vi "encoder_debug_v2.vi"() -> ()   [LabVIEW 2014]
uses:
  <vilib>/rvi/Emulation/niFpgaGetClockAttributes.vi
  <vilib>/rvi/Emulation/niFpgaSctlEmulationGetInTimedLoop.vi
  <vilib>/rvi/Emulation/niFpgaEmulationReportErrorSimple.vi
  <vilib>/rvi/Emulation/niFpgaProcessEmulError.vi
  <vilib>/rvi/interface/RandomDataEmulation/nirviRandomDataMultiElementFPGAFIFO.vi
  <instcachedir>/0/nirviRandomDataMultiElementFPGAFIFO_AD0CFC12EF974623A9C2E4184BC062B2.lvgen/nirviRandomDataMultiElementFPGAFIFO_AD0CFC12EF974623A9C2E4184BC062B2_010.vi
  <vilib>/rvi/interface/RandomDataEmulation/niFpgaRandomDataHandleErrors.vi
  <vilib>/rvi/Emulation/niFpgaCriticalErrorInLSC.vi
  <vilib>/rvi/eio/common/nirviEmuTemplateMethod_errors.vi
  <vilib>/rvi/DataTransferAndStorage/Container/XNode/niFpgaContainer.xnode
  <vilib>/rvi/interface/RandomDataEmulation/nirviRandomDataFpgaMultiElementTemplate.vi
  <vilib>/eio/EIONode/EIONode.xnode
  <vilib>/rvi/Analysis/measure/butterworth/XNode/niFpgaButterworthFilter.xnode
panel:
  in  "Stop motor":bool
  out "omega_p2 (rad/s)":fxp<+/-,36,13>
  out "Dp2_d (mm/s)":fxp<+/-,36,13>
  out "omega_p2 (Mavg)":fxp<+/-,36,14>
  out "Dp2_d (Mavg)":fxp<+/-,36,14>
  in  "mt0_p2":u32
  out "Dp2_d (Mavg w. f.)":fxp<+/-,36,14>
  out "Dp1_d (Mavg w. f.)":fxp<+/-,36,14>
  in  "Dp_d (Mavg) coeff.":i32[](array[numeric])=[946630756, 63555534]
  in  "Dy_d (Mavg) coeff.":i32[](array[numeric])=[946630756, 63555534]
  out "omega_p2 (Mavg w. f.)":fxp<+/-,36,14>
  in  "omega_y(Mavg) coeff.":i32[](array[numeric])=[946630756, 63555534]
  out "omega_p1 (Mavg w. f)":fxp<+/-,36,14>
  in  "omega_P(Mavg) coeff.":i32[](array[numeric])=[946630756, 63555534]
  out "Dp1_d (T)":fxp<+/-,36,13>
  out "omega_p1 (T)":fxp<+/-,36,13>
  out "Dp2_d (T)":fxp<+/-,36,13>
  out "omega_p2 (T)":fxp<+/-,36,13>
  out "mt_omega_p2":u32
  out "Encoder Position_p2":i32
  out "D_p2":fxp<+/-,32,7>
  out "rad_p2":fxp<+/-,36,15>
  out "D_p1":fxp<+/-,32,7>
  out "rad_p1":fxp<+/-,36,15>
  out "Encoder Position_p1":i32
  out "Dp1_d (Mavg)":fxp<+/-,36,14>
  out "omega_p1 (Mavg)":fxp<+/-,36,14>
  in  "Dp_d_M_avg_Tc (uSec)":i32
  in  "Vp. Est.":i16(ring) items=["T", "Mavg", "Mavg w. f."]
  in  "Mag. factor_p":fxp<+/-,20,3>
  in  "Belt_out_p":fxp<+/-,7,7>
  in  "Belt_in_p":fxp<+/-,6,6>
  in  "mt0_p1":u32
  out "Dp1_d (mm/s)":fxp<+/-,36,13>
  out "omega_p1 (rad/s)":fxp<+/-,36,13>
  out "mt_omega_p1":u32
  in  "Encoder reset_p":bool
  out "Time now(s)":fxp<+,52,14>
  in  "Ini coe.":bool
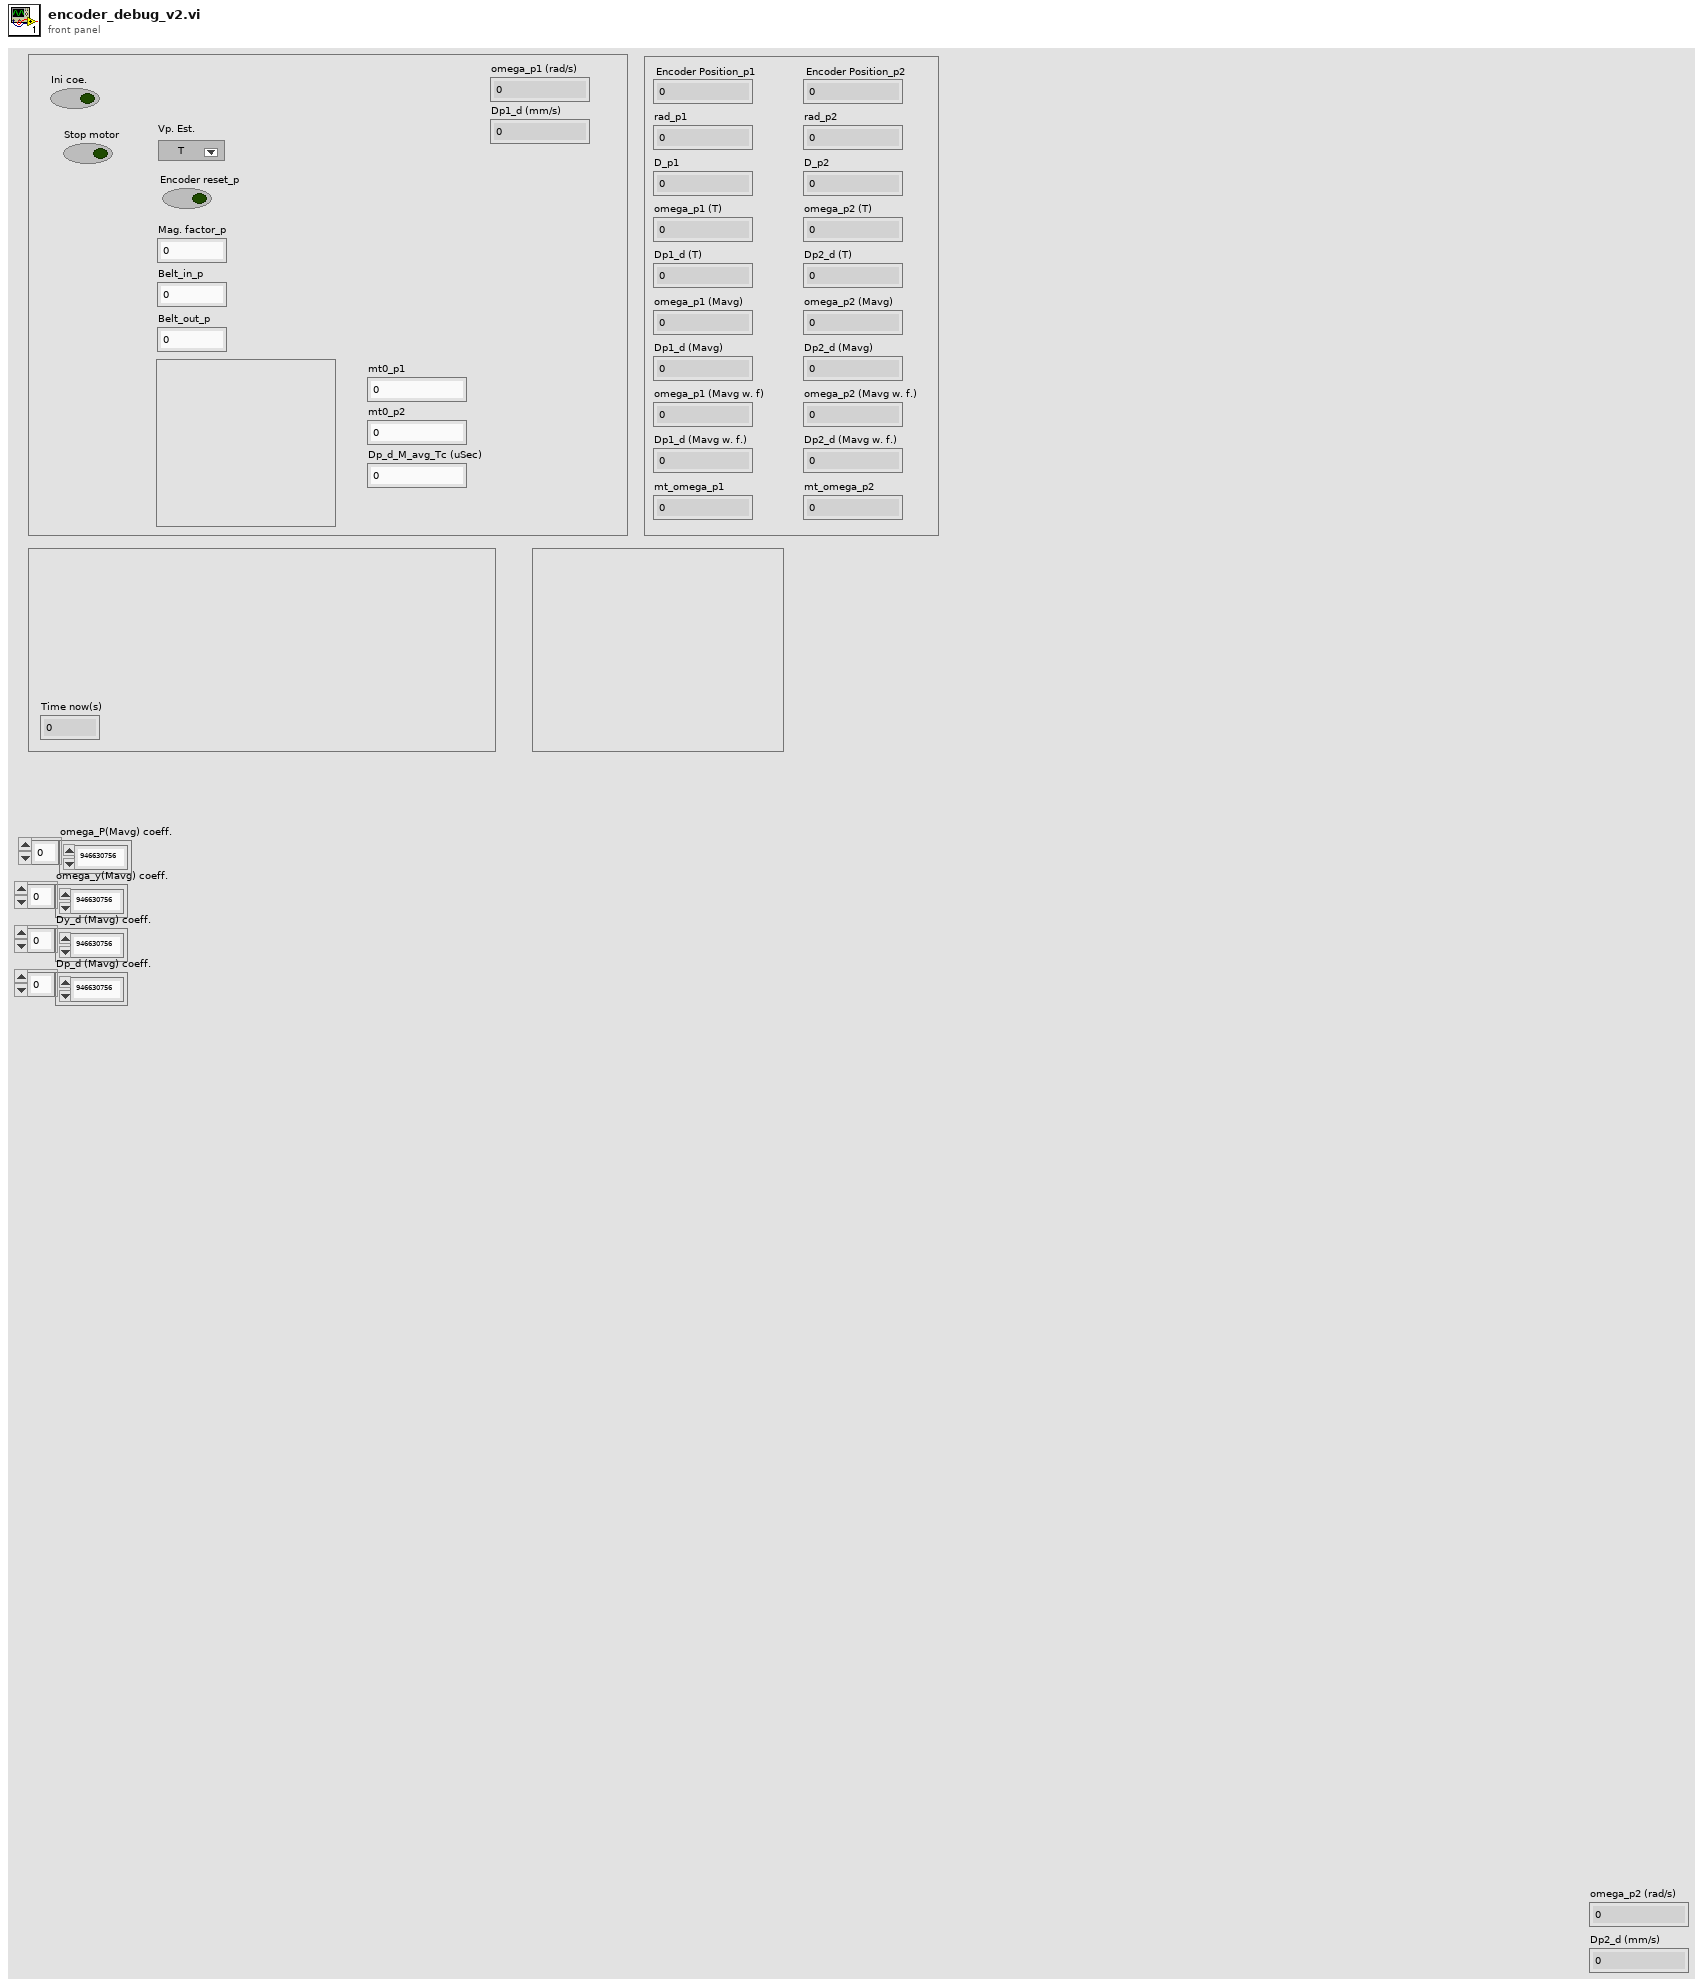
[diagram p1: front panel]
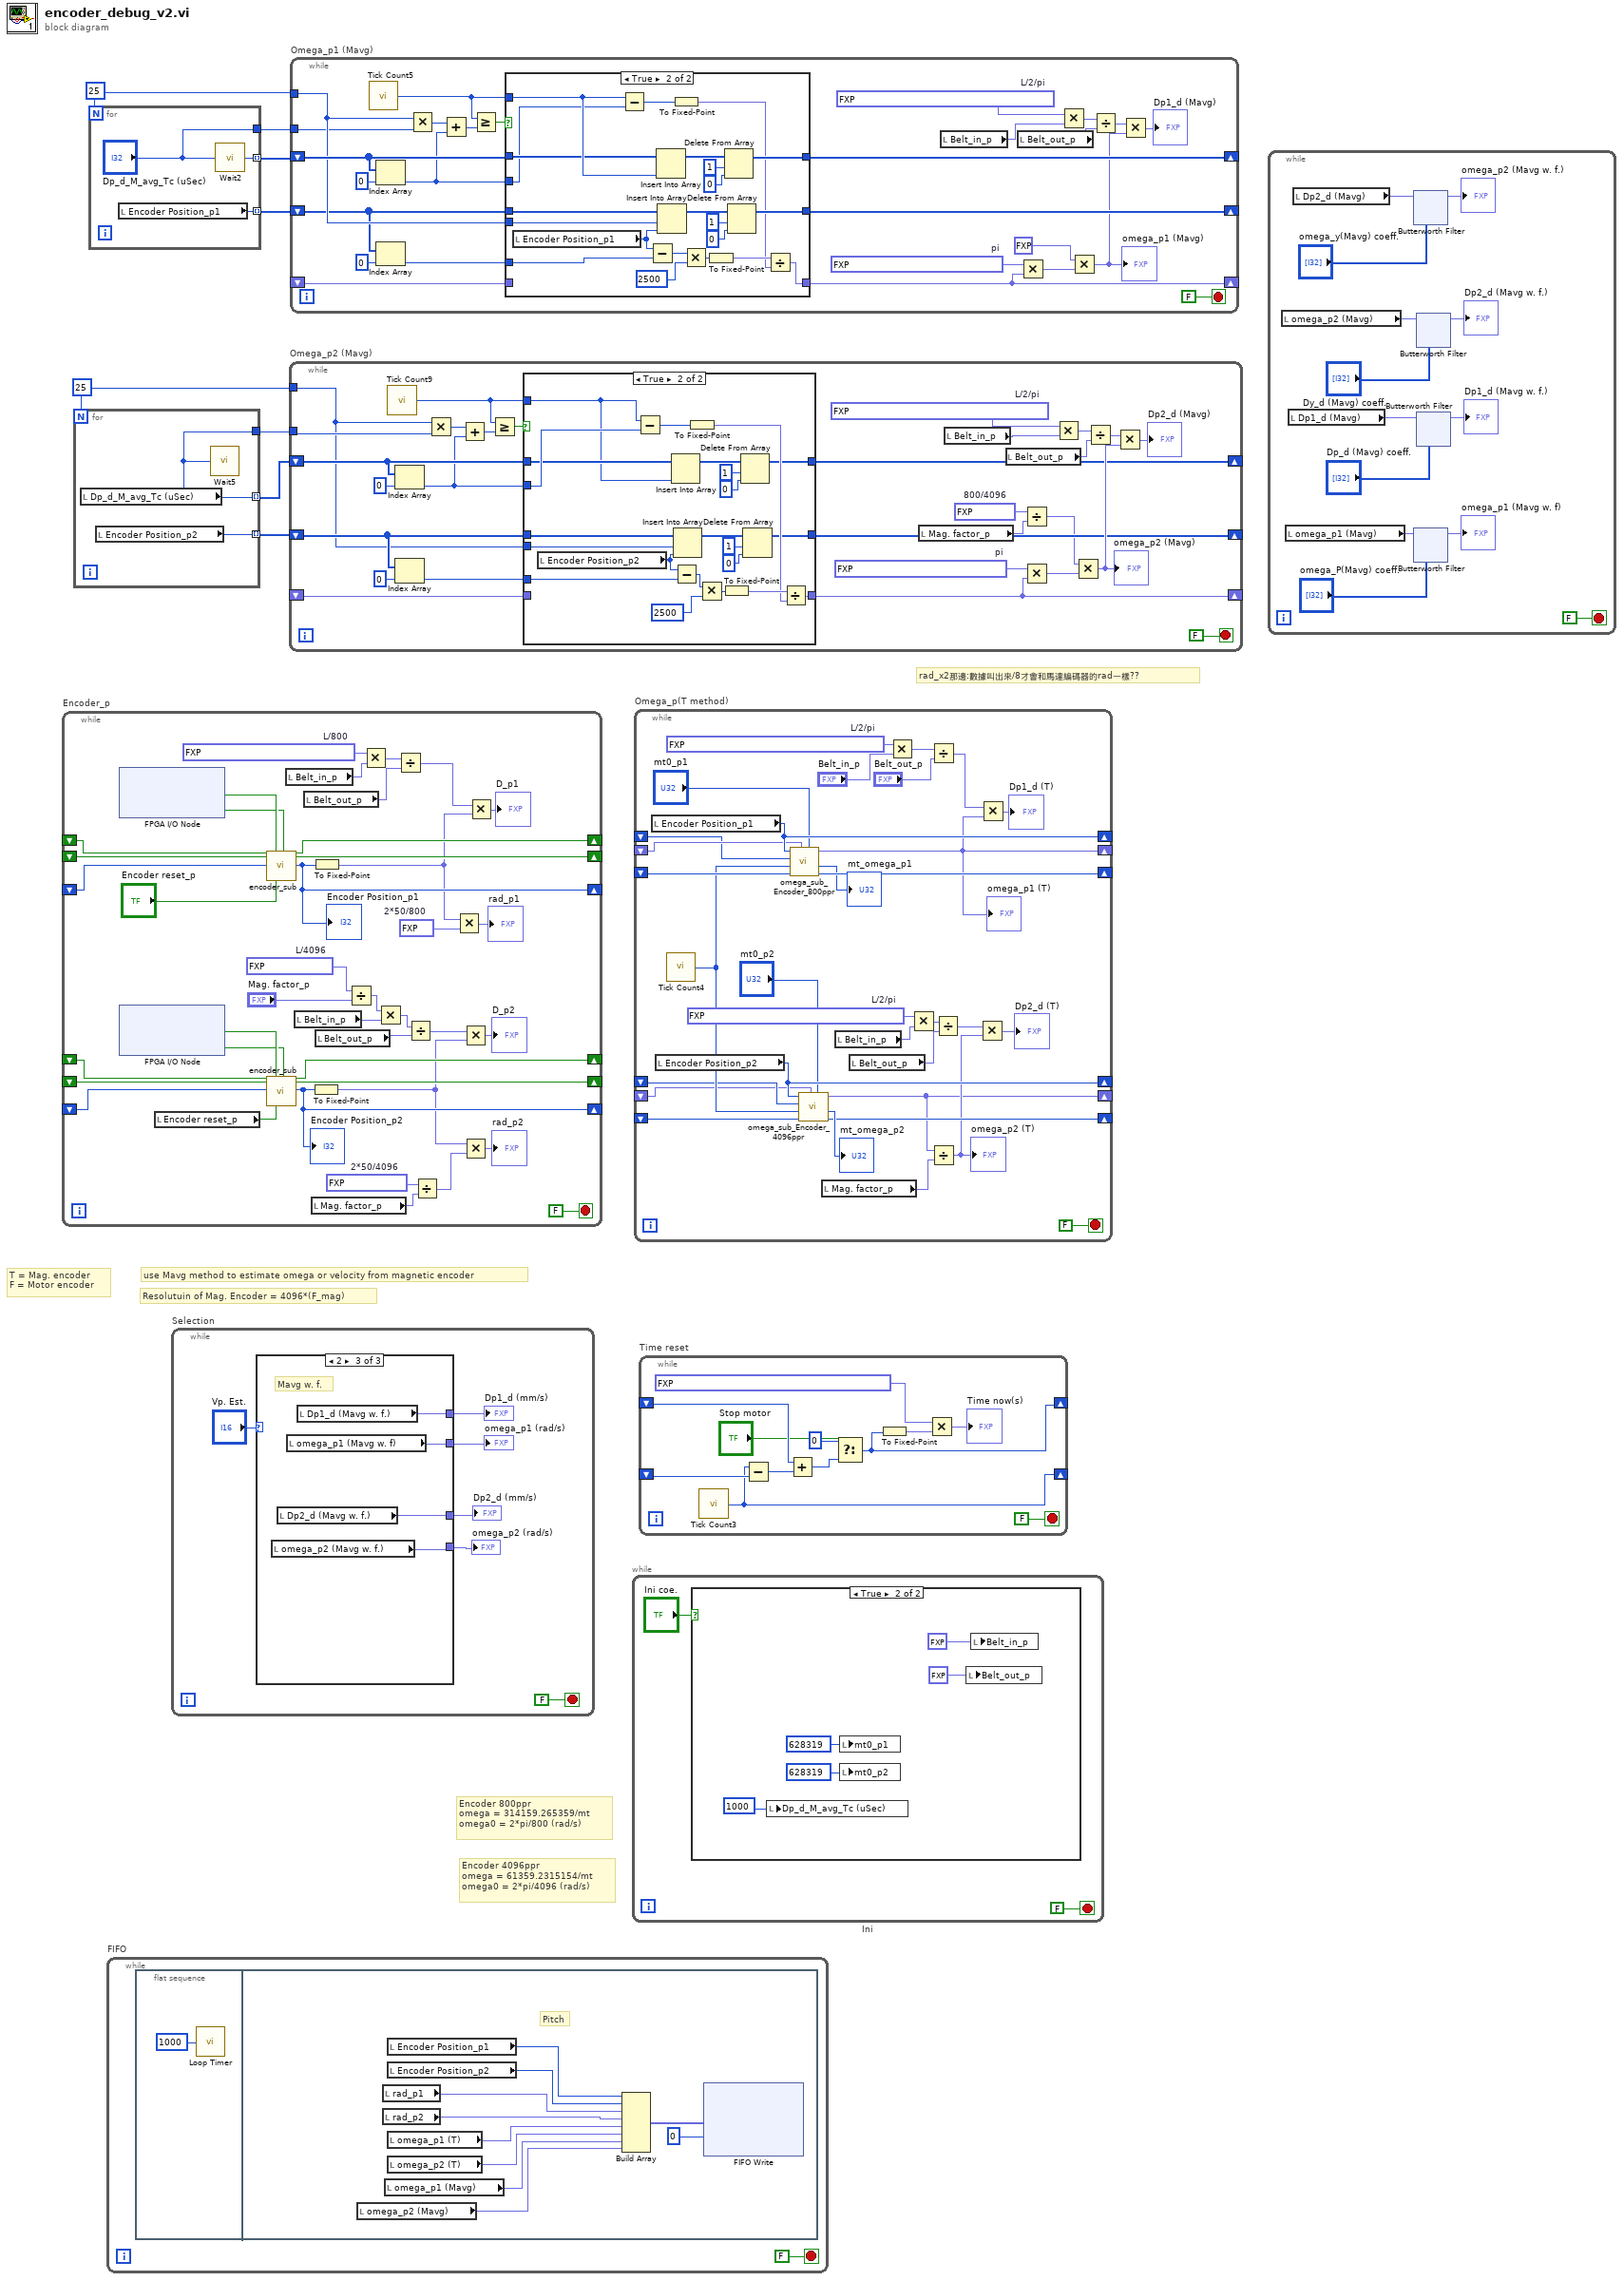
[diagram p0: block diagram]
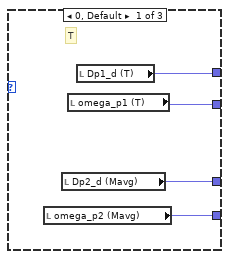
[diagram p4: hidden frame]
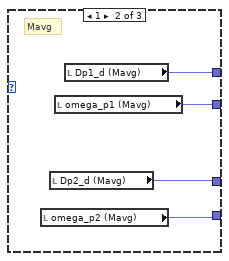
[diagram p5: hidden frame]
diagram:
  w2 = 25
  w8 = 25
  # "T = Mag. encoder\nF = Motor encoder"
  # "rad_x2那邊:數據叫出來/8才會和馬達編碼器的rad一樣??"
  # "Encoder 4096ppr\nomega = 61359.2315154/mt\nomega0 = 2*pi/4096 (rad/s)"
  # "Encoder 800ppr\nomega = 314159.265359/mt\nomega0 = 2*pi/800 (rad/s)"
  # "Resolutuin of Mag. Encoder = 4096*(F_mag)"
  # "use Mavg method to estimate omega or velocity from magnetic encoder"
  n1 = while "Encoder_p" {
    shift-right: [w46] -> _
    shift-left: _ -> [w45]
    shift-right: [w47] -> _
    shift-left: _ -> [w44]
    shift-right: [w41] -> _
    shift-left: _ -> [w43]
    shift-right: [w32] -> _
    shift-left: _ -> [w31]
    shift-right: [w33] -> _
    shift-left: _ -> [w34]
    shift-right: [w28] -> _
    shift-left: _ -> [w29]
    stop <- FALSE stop-if-true
    w24 = fxp<+/-,20,-5> 0.00048828125  # L/4096
    w22 = fxp<+/-,16,1> 0.0244140625  # 2*50/4096
    w40 = fxp<+/-,20,-5> 0.002499997615814209  # L/800
    w14 = fxp<+/-,16,1> 0.125  # 2*50/800
    n2 = xnode "FPGA I/O Node"() -> ("Mod7/DIO0"=w49:bool, "Mod7/DIO1"=w48:bool)  [unwired: 2 in, 2 out]
    n3 = xnode "FPGA I/O Node"() -> ("Mod7/DIO4"=w36:bool, "Mod7/DIO5"=w35:bool)  [unwired: 2 in, 2 out]
    n4 = local read "Encoder reset_p"() -> (w30:bool)
    n5 = call "encoder_sub.vi"("A_pre"=w45, "B_pre"=w44, "Encoder Position_pre"=w43, "A input"=w49, "Encoder Position Reset"="Encoder reset_p", "B input"=w48) -> ("A"=w46:bool, "B"=w47:bool, "Encoder Position (Counts)"=w41:i32)  [unwired: 19 in]
    "Encoder Position_p1" <- w41
    n6 = call "encoder_sub.vi"("A_pre"=w31, "B_pre"=w34, "Encoder Position_pre"=w29, "A input"=w36, "Encoder Position Reset"=w30, "B input"=w35) -> ("A"=w32:bool, "B"=w33:bool, "Encoder Position (Counts)"=w28:i32)  [unwired: 19 in]
    "Encoder Position_p2" <- w28
    n7 = local read "Belt_in_p"() -> (w39:fxp<+/-,6,6>)
    n8 = local read "Belt_in_p"() -> (w25:fxp<+/-,6,6>)
    n9 = local read "Belt_out_p"() -> (w37:fxp<+/-,7,7>)
    n10 = local read "Mag. factor_p"() -> (w21:fxp<+/-,20,3>)
    n11 = To Fixed-Point(number=w28) -> (fixed-point=w10:fxp<+/-,32,32>)  [unwired: 1 in]
    n12 = To Fixed-Point(number=w41) -> (fixed-point=w15:fxp<+/-,32,32>)  [unwired: 1 in]
    n13 = local read "Belt_out_p"() -> (w27:fxp<+/-,7,7>)
    n14 = Divide(x=w24, y="Mag. factor_p") -> (x/y=w23:fxp<+/-,41,13>)
    n15 = Multiply(x=w40, y=w39) -> (x*y=w38:fxp<+/-,26,1>)
    n16 = Multiply(x=w23, y=w25) -> (x*y=w26:fxp<+/-,46,18>)
    n17 = Divide(x=w38, y=w37) -> (x/y=w17:fxp<+/-,33,1>)
    n18 = Divide(x=w26, y=w27) -> (x/y=w12:fxp<+/-,53,18>)
    n19 = Divide(x=w22, y=w21) -> (x/y=w9:fxp<+/-,37,19>)
    n20 = Multiply(x=w15, y=w14) -> (x*y=→"rad_p1":fxp<+/-,48,33>)
    n21 = Multiply(x=w12, y=w10) -> (x*y=→"D_p2":fxp<+/-,64,49>)
    n22 = Multiply(x=w10, y=w9) -> (x*y=→"rad_p2":fxp<+/-,64,50>)
    n23 = Multiply(x=w17, y=w15) -> (x*y=→"D_p1":fxp<+/-,64,32>)
  }
  n24 = for {
    N: w2 -> [_]
    tunnel: [w51] -> w4 mode=indexing
    tunnel: [w50] -> w3 mode=indexing
    tunnel: [w50] -> w1
    n25 = local read "Dp_d_M_avg_Tc (uSec)"() -> (w50:i32)
    n26 = local read "Encoder Position_p2"() -> (w51:i32)
    n27 = call "Wait5"("Count(uSec)"=w50) -> ()  [unwired: 1 out]
  }
  n28 = for {
    N: w8 -> [_]
    tunnel: ["Dp_d_M_avg_Tc (uSec)"] -> w5
    tunnel: [w53] -> w7 mode=indexing
    tunnel: [w52] -> w6 mode=indexing
    n29 = local read "Encoder Position_p1"() -> (w52:i32)
    n30 = call "Wait2"("Count(uSec)"="Dp_d_M_avg_Tc (uSec)") -> ("Tick Count(uSec)"=w53:u32)
  }
  n31 = while "FIFO" {
    stop <- FALSE stop-if-true
    n32 = flat-sequence {
      frame #0 {
        n33 = call "Loop Timer"("Count(uSec)"=u32 1000) -> ()  [unwired: 1 out]
      }
      frame #1 {
        # "Pitch"
        n34 = local read "omega_p2 (Mavg)"() -> (w57:fxp<+/-,36,14>)
        n35 = local read "rad_p1"() -> (w64:fxp<+/-,36,15>)
        n36 = local read "rad_p2"() -> (w63:fxp<+/-,36,15>)
        n37 = local read "omega_p1 (Mavg)"() -> (w61:fxp<+/-,36,14>)
        n38 = local read "Encoder Position_p1"() -> (w66:i32)
        n39 = local read "Encoder Position_p2"() -> (w65:i32)
        n40 = local read "omega_p1 (T)"() -> (w59:fxp<+/-,36,13>)
        n41 = local read "omega_p2 (T)"() -> (w60:fxp<+/-,36,13>)
        n42 = Build Array(w66, w65, w64, w63, w59, w60, w61, w57) -> (w58:fxp<+/-,55,32>[])
        n43 = xnode ("FIFO Write")("Element"=w58, "Timeout"=0) -> ()  [unwired: 1 in, 2 out]
      }
    }
  }
  n44 = while "Selection" {
    stop <- FALSE stop-if-true
    n45 = case shown="2" "Vp. Est." {
      tunnel: [w76 w79 w84] -> w71
      tunnel: [w75 w80 w83] -> w72
      tunnel: [w74 w77 w81] -> w69
      tunnel: [w73 w78 w82] -> w68
      frame 0, Default {
        # "T"
        n46 = local read "omega_p2 (Mavg)"() -> (w74:fxp<+/-,36,14>)
        n47 = local read "Dp2_d (Mavg)"() -> (w73:fxp<+/-,36,14>)
        n48 = local read "omega_p1 (T)"() -> (w76:fxp<+/-,36,13>)
        n49 = local read "Dp1_d (T)"() -> (w75:fxp<+/-,36,13>)
      }
      frame 1 {
        # "Mavg"
        n50 = local read "omega_p2 (Mavg)"() -> (w77:fxp<+/-,36,14>)
        n51 = local read "Dp2_d (Mavg)"() -> (w78:fxp<+/-,36,14>)
        n52 = local read "omega_p1 (Mavg)"() -> (w79:fxp<+/-,36,14>)
        n53 = local read "Dp1_d (Mavg)"() -> (w80:fxp<+/-,36,14>)
      }
      frame 2 {
        # "Mavg w. f."
        n54 = local read "omega_p2 (Mavg w. f.)"() -> (w81:fxp<+/-,36,14>)
        n55 = local read "Dp2_d (Mavg w. f.)"() -> (w82:fxp<+/-,36,14>)
        n56 = local read "omega_p1 (Mavg w. f)"() -> (w84:fxp<+/-,36,14>)
        n57 = local read "Dp1_d (Mavg w. f.)"() -> (w83:fxp<+/-,36,14>)
      }
    }
    "Dp1_d (mm/s)" <- w72
    "omega_p1 (rad/s)" <- w71
    "Dp2_d (mm/s)" <- w68
    "omega_p2 (rad/s)" <- w69
  }
  n58 = while "Omega_p2 (Mavg)" {
    shift-right: [w86] -> _
    shift-left: w4 -> [w107]
    shift-right: [w87] -> _
    shift-left: w3 -> [w105]
    shift-right: [w91] -> _
    shift-left: _ -> [w89]
    tunnel: w2 -> [w103]
    tunnel: w1 -> [w108]
    stop <- FALSE stop-if-true
    w92 = fxp<+/-,27,3> 3.1415926814079285  # pi
    w95 = fxp<+,32,0> 0.1953125  # 800/4096
    w100 = fxp<+/-,32,0> 0.3183098859153688  # L/2/pi
    n59 = call "Tick Count9"() -> ("Tick Count(uSec)"=w102:u32)
    n60 = Index Array(array=w105, index=0) -> (element=w104:i32)
    n61 = Index Array(array=w107, index=0) -> (element=w106:i32)
    n62 = Multiply(x=w103, y=w108) -> (x*y=w111:i32)
    n63 = Add(x=w111, y=w104) -> (x+y=w110:i32)
    n64 = Greater Or Equal?(x=w102, y=w110) -> (x >= y?=w109:bool)
    n65 = case shown="True" w109 {
      tunnel: w107 -> [w115 w130]
      tunnel: w106 -> [_ w122]
      tunnel: w105 -> [w116 w131]
      tunnel: w104 -> [_ w132]
      tunnel: w103 -> [_ w129]
      tunnel: w102 -> [_ w117]
      tunnel: [w115 w120] -> w86
      tunnel: [w116 w119] -> w87
      tunnel: [w114 w118] -> w91
      tunnel: w89 -> [w114 _]
      frame False {
      }
      frame True {
        n66 = local read "Encoder Position_p2"() -> (w121:i32)
        n67 = Subtract(x=w117, y=w132) -> (x-y=w133:u32)
        n68 = Insert Into Array(array=w131, new element=w117) -> (w135:i32[])  [unwired: 1 in]
        n69 = Subtract(x=w121, y=w122) -> (x-y=w126:i32)
        n70 = Insert Into Array(array=w130, index=w129, new element=w121) -> (w136:i32[])
        n71 = To Fixed-Point(number=w133) -> (fixed-point=w123:fxp<+,32,32>)  [unwired: 1 in]
        n72 = Multiply(x=w126, y=2500) -> (x*y=w127:i32)
        n73 = To Fixed-Point(number=w127) -> (fixed-point=w128:fxp<+/-,32,32>)  [unwired: 1 in]
        n74 = Delete From Array(array=w135, length=1, index=0) -> (array with subset deleted=w119:i32[])  [unwired: 1 out]
        n75 = Delete From Array(array=w136, length=1, index=0) -> (array with subset deleted=w120:i32[])  [unwired: 1 out]
        n76 = Divide(x=w128, y=w123) -> (x/y=w118:fxp<+/-,64,32>)
      }
    }
    n77 = local read "Mag. factor_p"() -> (w94:fxp<+/-,20,3>)
    n78 = local read "Belt_in_p"() -> (w97:fxp<+/-,6,6>)
    n79 = local read "Belt_out_p"() -> (w96:fxp<+/-,7,7>)
    n80 = Divide(x=w95, y=w94) -> (x/y=w85:fxp<+/-,32,1>)
    n81 = Multiply(x=w92, y=w91) -> (x*y=w93:fxp<+/-,64,35>)
    n82 = Multiply(x=w100, y=w97) -> (x*y=w101:fxp<+/-,38,6>)
    n83 = Multiply(x=w85, y=w93) -> (x*y=w88:fxp<+/-,64,36>)
    "omega_p2 (Mavg)" <- w88
    n84 = Divide(x=w101, y=w96) -> (x/y=w99:fxp<+/-,45,6>)
    n85 = Multiply(x=w99, y=w88) -> (x*y=→"Dp2_d (Mavg)":fxp<+/-,64,41>)
  }
  n86 = while "Omega_p1 (Mavg)" {
    tunnel: w8 -> [w157]
    shift-right: [w155] -> _
    shift-left: w7 -> [w160]
    shift-right: [w154] -> _
    shift-left: w6 -> [w156]
    shift-right: [w153] -> _
    shift-left: _ -> [w152]
    tunnel: w5 -> [w150]
    stop <- FALSE stop-if-true
    w144 = fxp<+/-,27,3> 3.1415926814079285  # pi
    w143 = fxp<+/-,32,0> 0.3183098859153688  # L/2/pi
    n87 = call "Tick Count5"() -> ("Tick Count(uSec)"=w161:u32)
    n88 = Index Array(array=w160, index=0) -> (element=w159:u32)
    n89 = Index Array(array=w156, index=0) -> (element=w158:i32)
    n90 = Multiply(x=w157, y=w150) -> (x*y=w163:i32)
    n91 = Add(x=w163, y=w159) -> (x+y=w162:u32)
    n92 = Greater Or Equal?(x=w161, y=w162) -> (x >= y?=w151:bool)
    n93 = case shown="True" w151 {
      tunnel: w161 -> [_ w184]
      tunnel: w157 -> [_ w181]
      tunnel: w160 -> [w168 w183]
      tunnel: w159 -> [_ w182]
      tunnel: w158 -> [_ w178]
      tunnel: w156 -> [w167 w180]
      tunnel: [w166 w176] -> w153
      tunnel: [w168 w175] -> w155
      tunnel: [w167 w174] -> w154
      tunnel: w152 -> [w166 _]
      frame False {
      }
      frame True {
        n94 = local read "Encoder Position_p1"() -> (w177:i32)
        n95 = Subtract(x=w184, y=w182) -> (x-y=w185:u32)
        n96 = Subtract(x=w177, y=w178) -> (x-y=w170:i32)
        n97 = Insert Into Array(array=w183, new element=w184) -> (w187:u32[])  [unwired: 1 in]
        n98 = Insert Into Array(array=w180, index=w181, new element=w177) -> (w188:i32[])
        n99 = To Fixed-Point(number=w185) -> (fixed-point=w172:fxp<+,32,32>)  [unwired: 1 in]
        n100 = Multiply(x=w170, y=2500) -> (x*y=w171:i32)
        n101 = To Fixed-Point(number=w171) -> (fixed-point=w179:fxp<+/-,32,32>)  [unwired: 1 in]
        n102 = Delete From Array(array=w187, length=1, index=0) -> (array with subset deleted=w175:u32[])  [unwired: 1 out]
        n103 = Delete From Array(array=w188, length=1, index=0) -> (array with subset deleted=w174:i32[])  [unwired: 1 out]
        n104 = Divide(x=w179, y=w172) -> (x/y=w176:fxp<+/-,64,32>)
      }
    }
    n105 = local read "Belt_in_p"() -> (w148:fxp<+/-,6,6>)
    n106 = local read "Belt_out_p"() -> (w147:fxp<+/-,7,7>)
    n107 = Multiply(x=w144, y=w153) -> (x*y=w149:fxp<+/-,64,35>)
    n108 = Multiply(x=w143, y=w148) -> (x*y=w146:fxp<+/-,38,6>)
    n109 = Multiply(x=fxp<+/-,2,2> 1.0 ("f"), y=w149) -> (x*y=w142:fxp<+/-,64,37>)
    "omega_p1 (Mavg)" <- w142
    n110 = Divide(x=w146, y=w147) -> (x/y=w141:fxp<+/-,45,6>)
    n111 = Multiply(x=w141, y=w142) -> (x*y=→"Dp1_d (Mavg)":fxp<+/-,64,42>)
  }
  n112 = while "Ini" {
    stop <- FALSE stop-if-true
    n113 = case shown="True" "Ini coe." {
      frame False {
      }
      frame True {
        n114 = local write "Dp_d_M_avg_Tc (uSec)"(u32 1000 ("D_d_M_avg_Tc (uSec)")) -> ()
        n115 = local write "mt0_p1"(u32 628319 ("mt0_p1")) -> ()
        n116 = local write "mt0_p2"(u32 628319 ("mt0_p2")) -> ()
        n117 = local write "Belt_out_p"(fxp<+/-,7,7> 36.0 ("Belt_op")) -> ()
        n118 = local write "Belt_in_p"(fxp<+/-,6,6> 14.0 ("Belt_mp")) -> ()
      }
    }
  }
  n119 = while "Omega_p(T method)" {
    shift-right: [w229] -> _
    shift-left: _ -> [w227]
    shift-right: [w210] -> _
    shift-left: _ -> [w228]
    shift-right: [w225] -> _
    shift-left: _ -> [w226]
    shift-right: [w203] -> _
    shift-left: _ -> [w202]
    shift-right: [w198] -> _
    shift-left: _ -> [w200]
    shift-right: [w206] -> _
    shift-left: _ -> [w205]
    stop <- FALSE stop-if-true
    w217 = fxp<+/-,32,0> 0.3183098859153688  # L/2/pi
    w222 = fxp<+/-,32,0> 0.3183098859153688  # L/2/pi
    n120 = local read "Encoder Position_p1"() -> (w229:i32)
    n121 = local read "Encoder Position_p2"() -> (w203:i32)
    n122 = call "Tick Count4"() -> ("Tick Count(Ticks)"=w204:u32)
    n123 = call "omega_sub_Encoder_800ppr.vi"("mt0"="mt0_p1", "omega_pre"=w228, "ticks_m_pre"=w226, "ticks"=w204, "count_pre"=w227, "count"=w229) -> ("ticks_m"=w225:u32, "mt"=→"mt_omega_p1":u32, "omega"=w210:fxp<+/-,36,13>)  [unwired: 3 in]
    "omega_p1 (T)" <- w210
    n124 = call "omega_sub_Encoder_4096ppr.vi"("mt0"="mt0_p2", "omega_pre"=w200, "ticks_m_pre"=w205, "ticks"=w204, "count_pre"=w202, "count"=w203) -> ("ticks_m"=w206:u32, "mt"=→"mt_omega_p2":u32, "omega"=w198:fxp<+/-,36,13>)  [unwired: 3 in]
    n125 = local read "Mag. factor_p"() -> (w218:fxp<+/-,20,3>)
    n126 = local read "Belt_in_p"() -> (w215:fxp<+/-,6,6>)
    n127 = local read "Belt_out_p"() -> (w214:fxp<+/-,7,7>)
    n128 = Multiply(x=w222, y="Belt_in_p") -> (x*y=w220:fxp<+/-,38,6>)
    n129 = Multiply(x=w217, y=w215) -> (x*y=w216:fxp<+/-,38,6>)
    n130 = Divide(x=w220, y="Belt_out_p") -> (x/y=w211:fxp<+/-,20,1>)
    n131 = Divide(x=w198, y=w218) -> (x/y=w199:fxp<+/-,57,31>)
    "omega_p2 (T)" <- w199
    n132 = Divide(x=w216, y=w214) -> (x/y=w209:fxp<+/-,45,6>)
    n133 = Multiply(x=w209, y=w199) -> (x*y=→"Dp2_d (T)":fxp<+/-,36,13>)
    n134 = Multiply(x=w211, y=w210) -> (x*y=→"Dp1_d (T)":fxp<+/-,36,13>)
  }
  n135 = while "Time reset" {
    shift-right: [w240] -> _
    shift-left: _ -> [w241]
    shift-right: [w235] -> _
    shift-left: _ -> [w236]
    stop <- FALSE stop-if-true
    n136 = call "Tick Count3"() -> ("Tick Count(uSec)"=w240:u32)
    n137 = Subtract(x=w240, y=w241) -> (x-y=w239:u32)
    n138 = Add(x=w236, y=w239) -> (x+y=w238:u32)
    n139 = Select(t=u32 0, s="Stop motor", f=w238) -> (s? t:f=w235:u32)
    n140 = To Fixed-Point(number=w235) -> (fixed-point=w234:fxp<+,32,32>)  [unwired: 1 in]
    n141 = Multiply(x=fxp<+,20,-18> 1.0000003385357559e-06, y=w234) -> (x*y=→"Time now(s)":fxp<+,52,14>)
  }
  n142 = while {
    stop <- FALSE stop-if-true
    n143 = local read "omega_p2 (Mavg)"() -> (w247:fxp<+/-,36,14>)
    n144 = local read "omega_p1 (Mavg)"() -> (w254:fxp<+/-,36,14>)
    n145 = local read "Dp1_d (Mavg)"() -> (w246:fxp<+/-,36,14>)
    n146 = local read "Dp2_d (Mavg)"() -> (w250:fxp<+/-,36,14>)
    n147 = xnode "Butterworth Filter"("input data"=w250, "scaled coefficients"="omega_y(Mavg) coeff.") -> ("output data"=→"omega_p2 (Mavg w. f.)":fxp<+/-,36,18>)  [unwired: 1 in]
    n148 = xnode "Butterworth Filter"("input data"=w254, "scaled coefficients"="omega_P(Mavg) coeff.") -> ("output data"=→"omega_p1 (Mavg w. f)":fxp<+/-,36,18>)  [unwired: 1 in]
    n149 = xnode "Butterworth Filter"("input data"=w247, "scaled coefficients"="Dy_d (Mavg) coeff.") -> ("output data"=→"Dp2_d (Mavg w. f.)":fxp<+/-,36,18>)  [unwired: 1 in]
    n150 = xnode "Butterworth Filter"("input data"=w246, "scaled coefficients"="Dp_d (Mavg) coeff.") -> ("output data"=→"Dp1_d (Mavg w. f.)":fxp<+/-,36,18>)  [unwired: 1 in]
  }
